vi "(TestVI)example_get fw version.vi"() -> ()   [LabVIEW 2020]
uses:
  Controls/(Ctrl)Serial_FGV Function.ctl
panel:
  out "BD FW Version":u32 format="%08x"
  out "BD Version":enum8{"BBB 1.0", "BBB 1.1", "WBB 1.0"}(ring)
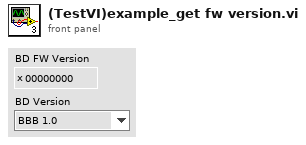
[diagram p1: front panel]
types:
  T1 = typedef "(Ctrl)Serial_FGV Function.ctl" = enum16{"Initialize", "Read", "Read All", "Write", "Flush Buffer", "Get Ref.", "Close"}
  T2 = enum8{"BBB 1.0", "BBB 1.1", "WBB 1.0", "reserved", "RedNoah3"}
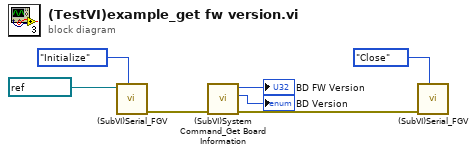
[diagram p0: block diagram]
diagram:
  n1 = call "(SubVI)Serial_FGV.vi"("Function"=(Ctrl)Serial_FGV_Function."Initialize", "VISA resource name"=refnum<visa-resource-name> "COM3") -> ("error out"=w6:errorcluster)  [unwired: 7 in, 2 out]
  n2 = call "(SubVI)System Command_Get Board Information.vi"("error in (no error)"=w6) -> ("error out"=w5:errorcluster, "BD HW Version"=→"BD Version":T2, "BD FW Version"=→"BD FW Version":u32)  [unwired: 3 in, 5 out]
  n3 = call "(SubVI)Serial_FGV.vi"("Function"=(Ctrl)Serial_FGV_Function."Close", "error in (no error)"=w5) -> ()  [unwired: 7 in, 3 out]
